vi "_PC_Toolbar_Set_Layout.vi"(5 "MachineType":enum16{"None", "MALDI", "ESI"}(ring), 6 "TagArray":string[](array[string])=["TIC", "System", "Recipe", "MS Periphery", "MS Cmd", "Advance"], 7 "Init?(F)":bool, 8 "error in (no error)":errorcluster, 10 "PanelRef_Array":refnum<vi>[](array[refnum]), 11 "SplitterRef_Array":refnum<vi>[](array[refnum])) -> (0 "error out":errorcluster)   [LabVIEW 2018]
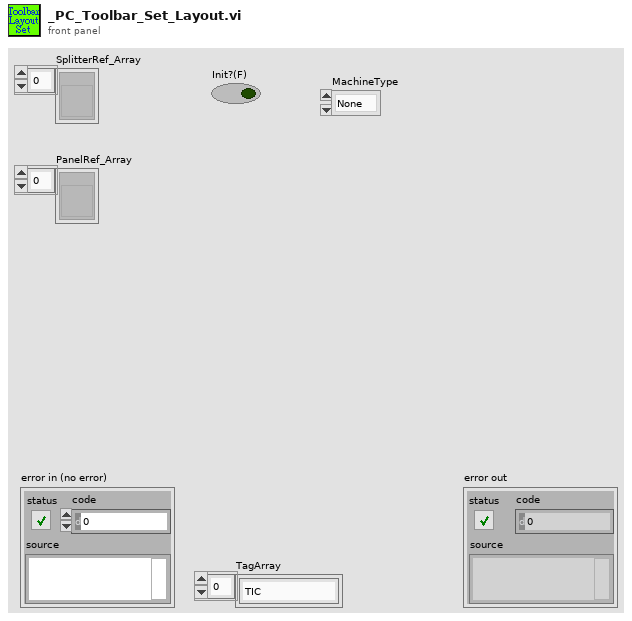
[diagram p1: front panel]
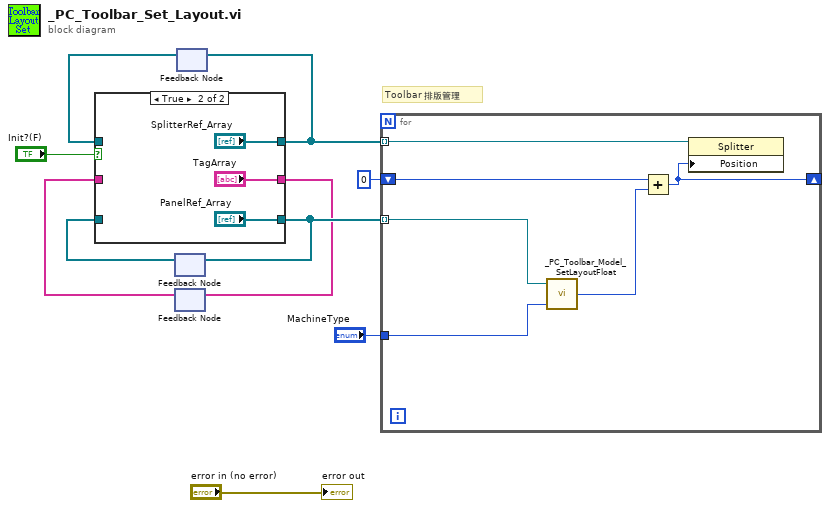
[diagram p0: block diagram]
diagram:
  # "Toolbar 排版管理"
  n1 = feedback #1() -> (w4:refnum<vi>[])  [unwired: 1 in]
  n2 = feedback #2() -> (w2:string[])  [unwired: 1 in]
  n3 = feedback #3() -> (w7:refnum<vi>[])  [unwired: 1 in]
  n4 = case shown="True" "Init?(F)" {
    tunnel: [w12 "SplitterRef_Array"] -> w6
    tunnel: [w13 "PanelRef_Array"] -> w5
    tunnel: w7 -> [w12 _]
    tunnel: w4 -> [w13 _]
    tunnel: [w11 "TagArray"] -> w3
    tunnel: w2 -> [w11 _]
    frame False {
    }
    frame True {
    }
  }
  n5 = feedback-in #1(w5) -> ()
  n6 = feedback-in #2(w3) -> ()
  n7 = feedback-in #3(w6) -> ()
  n8 = for {
    tunnel: w5 -> [w17] mode=indexing
    tunnel: w6 -> [w22] mode=indexing
    shift-right: [w19] -> _
    shift-left: 0 -> [w21]
    tunnel: "MachineType" -> [w18]
    n9 = call "_PC_Toolbar_Model_SetLayoutFloat.vi"("MachineType"=w18, "ToolBar_Panel_Ref"=w17) -> ("TotalWidth"=w20:i32)  [unwired: 1 in]
    n10 = Add(x=w21, y=w20) -> (x+y=w19:i32)
    n11 = property class="Splitter"(reference=w22, "Position"=w19) -> ()  [unwired: 1 in, 2 out]
  }
  "error out" <- "error in (no error)"
